vi "fp display engine resonance.vi"(7 "channel data in":sgl[][][](array[numeric]), 10 "Image Refs In":T1[](array[typedef]), 11 "DisplayRefsIn(generic class)":refnum<vi>[](array[refnum])) -> ()   [LabVIEW 2012]
doc: "SciScan 1.2 160622"
uses:
  <vilib>/vision/Image Controls.llb/IMAQ Image.ctl
  Custom Controls/MAIN Image panel reso tab Control type def.ctl
  Custom Controls/Image Types.ctl
  Custom Controls/Ch selector.ctl
  GFG/GFGbooleanGet.vi
  GFG/GFGfpRefGet.vi
  <vilib>/vision/NI_Vision_Development_Module.lvlib
  GFG/GFG library.lvlib
panel:
  in  "ROI colors":u32[](array[colorbox])=[6618880, 16716362, 16860, 16776793, 16750848, 16448250, 16716530, 9567230, 16764108, 7340212, 32639, 0, 13816530, 8421376, 8421631, 7171459, 6618880, 16716362, 16860, 16776793, 16750848, 16448250, 16716530, 9567230, 16764108, 7340212, 32639, 0, 13816530, 8421376, 8421631, 7171459, 6618880, 16716362, 16860, 16776793, 16750848, 16448250, 16716530, 9567230, 16764108, 7340212, 32639, 0, 13816530, 8421376, 8421631, 7171459, 6618880, 16716362, 16860, 16776793, 16750848, 16448250, 16716530, 9567230, 16764108, 7340212, 32639, 0, 13816530, 8421376, 8421631, 7171459, 6618880, 16716362, 16860, 16776793, 16750848, 16448250, 16716530, 9567230, 16764108, 7340212, 32639, 0, 13816530, 8421376, 8421631, 7171459, 6618880, 16716362, 16860, 16776793, 16750848, 16448250, 16716530, 9567230, 16764108, 7340212, 32639, 0, 13816530, 8421376, 8421631, 7171459, 6618880, 16716362, 16860, 16776793, 16750848, 16448250, 16716530, 9567230, 16764108, 7340212, 32639, 0, 13816530, 8421376, 8421631, 7171459, 6618880, 16716362, 16860, 16776793, 16750848, 16448250, 16716530, 9567230, 16764108, 7340212, 32639, 0, 13816530, 8421376, 8421631, 7171459, 6618880, 16716362, 16860, 16776793, 16750848, 16448250, 16716530, 9567230, 16764108, 7340212, 32639, 0, 13816530, 8421376, 8421631, 7171459, 6618880, 16716362, 16860, 16776793, 16750848, 16448250, 16716530, 9567230, 16764108, 7340212, 32639, 0, 13816530, 8421376, 8421631, 7171459, 6618880, 16716362, 16860, 16776793, 16750848, 16448250, 16716530, 9567230, 16764108, 7340212, 32639, 0, 13816530, 8421376, 8421631, 7171459, 6618880, 16716362, 16860, 16776793, 16750848, 16448250, 16716530, 9567230, 16764108, 7340212, 32639, 0, 13816530, 8421376, 8421631, 7171459, 6618880, 16716362, 16860, 16776793, 16750848, 16448250, 16716530, 9567230, 16764108, 7340212, 32639, 0, 13816530, 8421376, 8421631, 7171459, 6618880, 16716362, 16860, 16776793, 16750848, 16448250, 16716530, 9567230, 16764108, 7340212, 32639, 0, 13816530, 8421376, 8421631, 7171459, 6618880, 16716362, 16860, 16776793, 16750848, 16448250, 16716530, 9567230, 16764108, 7340212, 32639, 0, 13816530, 8421376, 8421631, 7171459, 6618880, 16716362, 16860, 16776793, 16750848, 16448250, 16716530, 9567230, 16764108, 7340212, 32639, 0, 13816530, 8421376, 8421631, 7171459, 6618880, 16716362, 16860, 16776793, 16750848, 16448250, 16716530, 9567230, 16764108, 7340212, 32639, 0, 13816530, 8421376, 8421631, 7171459, 6618880, 16716362, 16860, 16776793, 16750848, 16448250, 16716530, 9567230, 16764108, 7340212, 32639, 0, 13816530, 8421376, 8421631, 7171459, 6618880, 16716362, 16860, 16776793, 16750848, 16448250, 16716530, 9567230, 16764108, 7340212, 32639, 0, 13816530, 8421376, 8421631, 7171459, 6618880, 16716362, 16860, 16776793, 16750848, 16448250, 16716530, 9567230, 16764108, 7340212, 32639, 0, 13816530, 8421376, 8421631, 7171459, 6618880, 16716362, 16860, 16776793, 16750848, 16448250, 16716530, 9567230, 16764108, 7340212, 32639, 0, 13816530, 8421376, 8421631, 7171459, 6618880, 16716362, 16860, 16776793, 16750848, 16448250, 16716530, 9567230, 16764108, 7340212, 32639, 0, 13816530, 8421376, 8421631, 7171459, 6618880, 16716362, 16860, 16776793, 16750848, 16448250, 16716530, 9567230, 16764108, 7340212, 32639, 0, 13816530, 8421376, 8421631, 7171459, 6618880, 16716362, 16860, 16776793, 16750848, 16448250, 16716530, 9567230, 16764108, 7340212, 32639, 0, 13816530, 8421376, 8421631, 7171459, 6618880, 16716362, 16860, 16776793, 16750848, 16448250, 16716530, 9567230, 16764108, 7340212, 32639, 0, 13816530, 8421376, 8421631, 7171459]
  out "error out":errorcluster
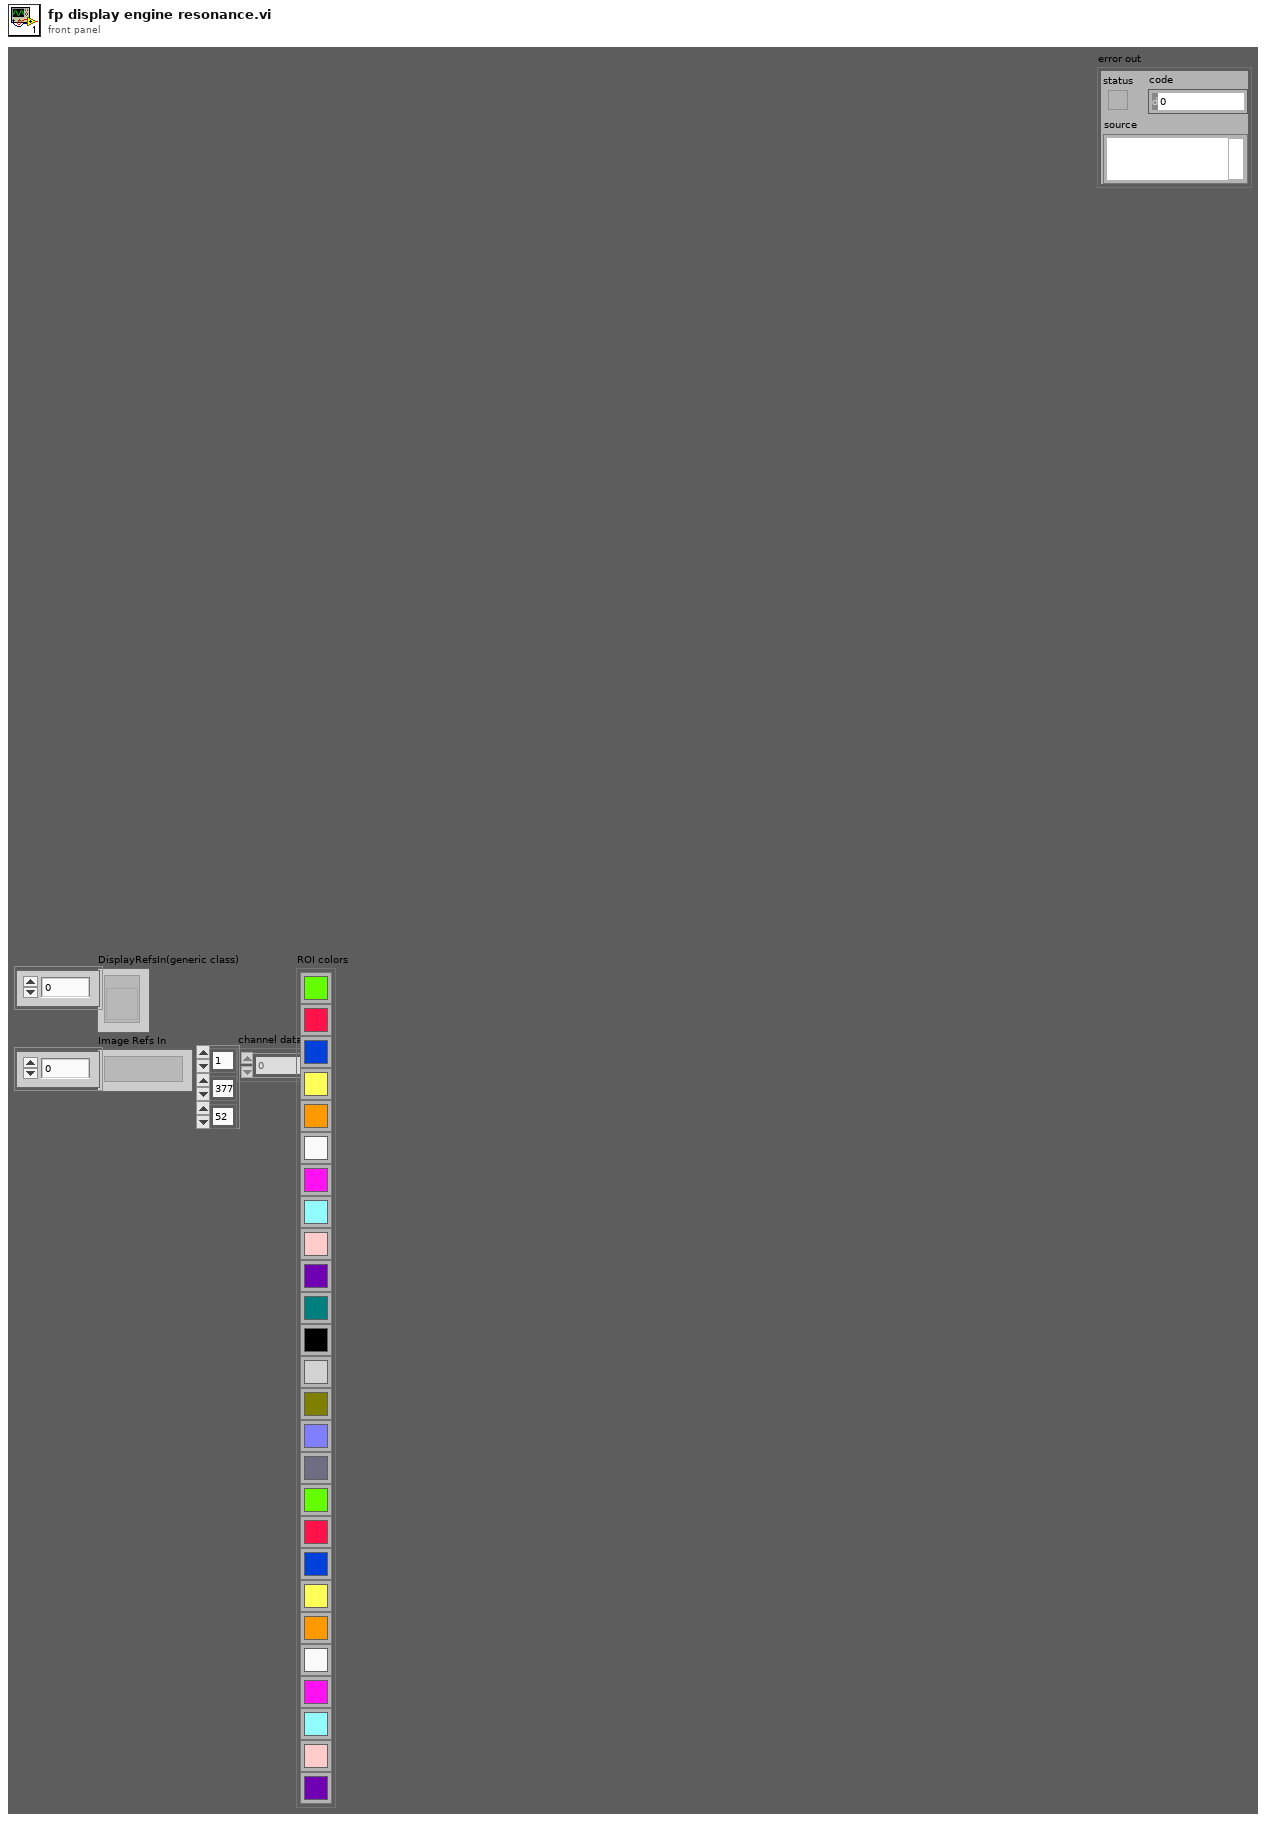
[diagram p1: front panel]
types:
  T1 = typedef "IMAQ Image.ctl" = refnum<image>
  T2 = typedef "MAIN Image panel reso tab Control type def.ctl" = enum32{"Channel 1", "Channel 2", "Channel 3", "Channel 4", "Channel 5", "all channels", "RGB overlay", "ROI", "arbitrary line scan"}
  T3 = enum32{"Channel 1", "Channel 2", "Channel 3", "Channel 4", "Channel 5", "all channels", "RGB overlay", "ROI", "arbitrary line scan"}
  T4 = typedef "Image Types.ctl" = enum16{"Frame Scan", "Line Scan", "RGB Overlay", "ROI", "All Channels Frame"}
  T5 = typedef "Ch selector.ctl" = enum16{"none", "Ch 1", "Ch 2", "Ch 3", "Ch 4"}
  T6 = typedef "Image Type" = u32
  T7 = cluster{"Global Rectangle":i32[], "Contours":cluster{"Contour Type":u32, "ROI Type":u32, "Points":i32[]}[]}
  T8 = typedef "ROI Descriptor" = cluster{"Global Rectangle":i32[], "Contours":cluster{"ID":enum32{"External", "Internal"}, "Type":u32, "Coordinates":i32[]}[]}
  T9 = cluster{"WaveformChartRef":refnum<vi>, "DigitalRef":refnum<vi>, "ArrayRef":refnum<vi>, "TabControlRef":refnum<vi>, "EnumRef":refnum<vi>, "RingRef":refnum<vi>, "BooleanRef":refnum<vi>, "KnobRef":refnum<vi>, "SlideRef":refnum<vi>, "PathRef":refnum<vi>, "StringRef":refnum<vi>, "ComboBox":refnum<vi>, "WaveformGraphRef":refnum<vi>}
  T10 = cluster{"Mean Value":sgl, "Standard Variation":sgl, "Minimal Value":sgl, "Maximal Value":sgl, "Area (calibrated)":sgl, "Area (pixels)":i32, "%":sgl}[]
  T11 = cluster{"Mean Value":sgl, "Standard Variation":sgl, "Minimal Value":sgl, "Maximal Value":sgl, "Area (calibrated)":sgl, "Area (pixels)":i32, "%":sgl}
  T12 = cluster{"Contour Type":u32, "ROI Type":u32, "Points":i32[]}[]
  T13 = cluster{"Starting Value":sgl, "Incremental Value":sgl, "Histogram":u32[]}
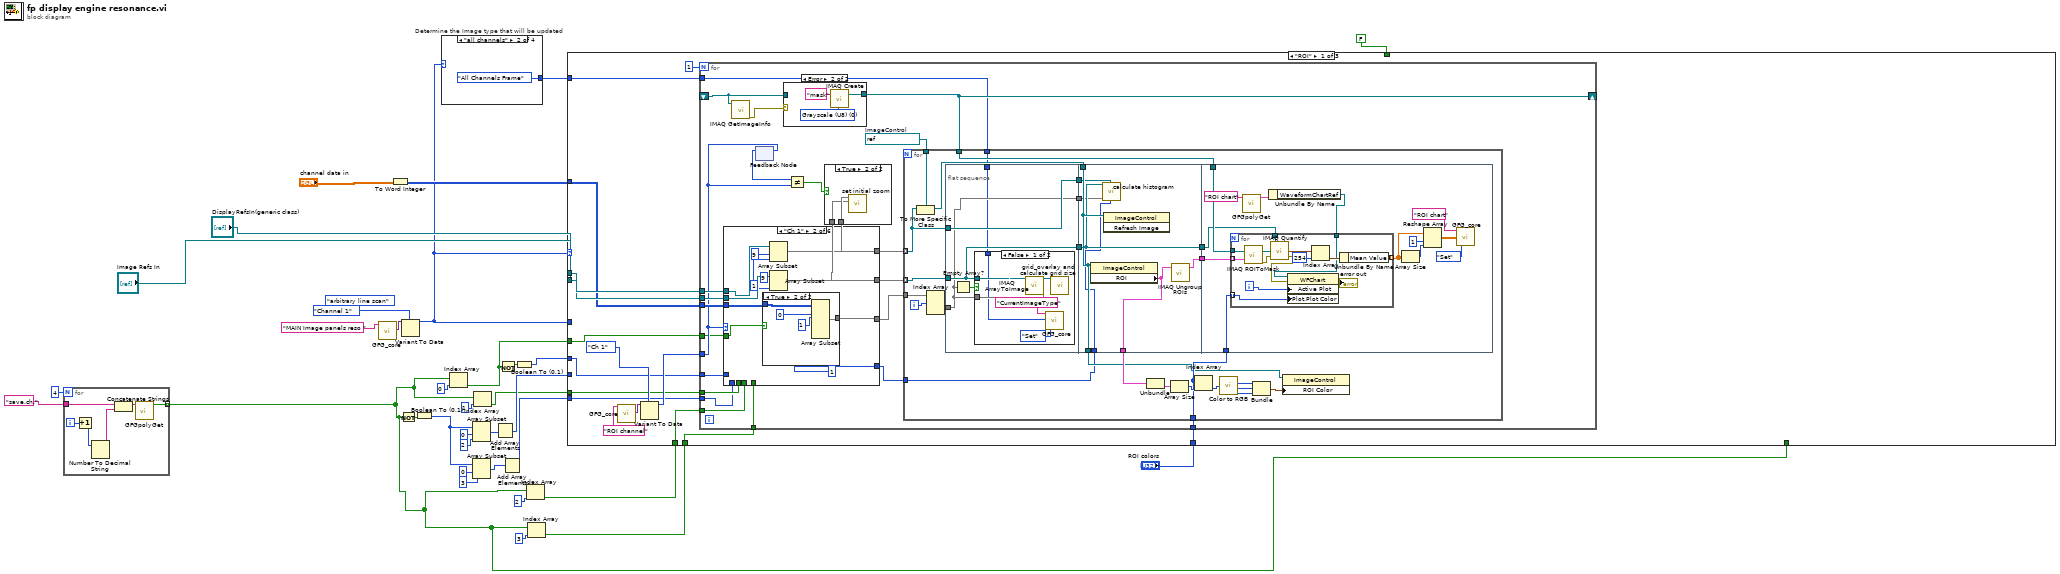
[diagram p0: block diagram]
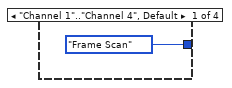
[diagram p2: hidden frame]
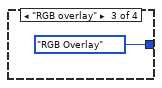
[diagram p3: hidden frame]
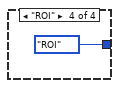
[diagram p4: hidden frame]
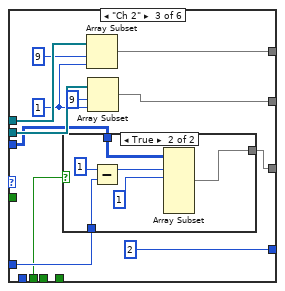
[diagram p9: hidden frame]
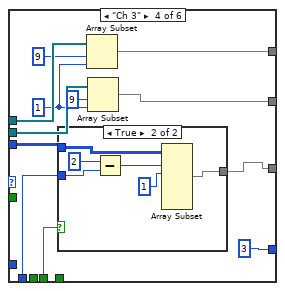
[diagram p11: hidden frame]
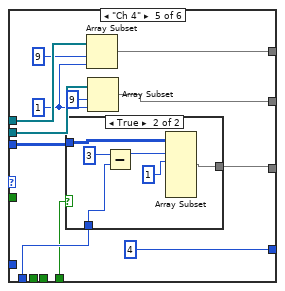
[diagram p13: hidden frame]
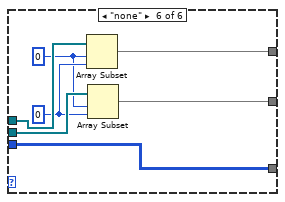
[diagram p15: hidden frame]
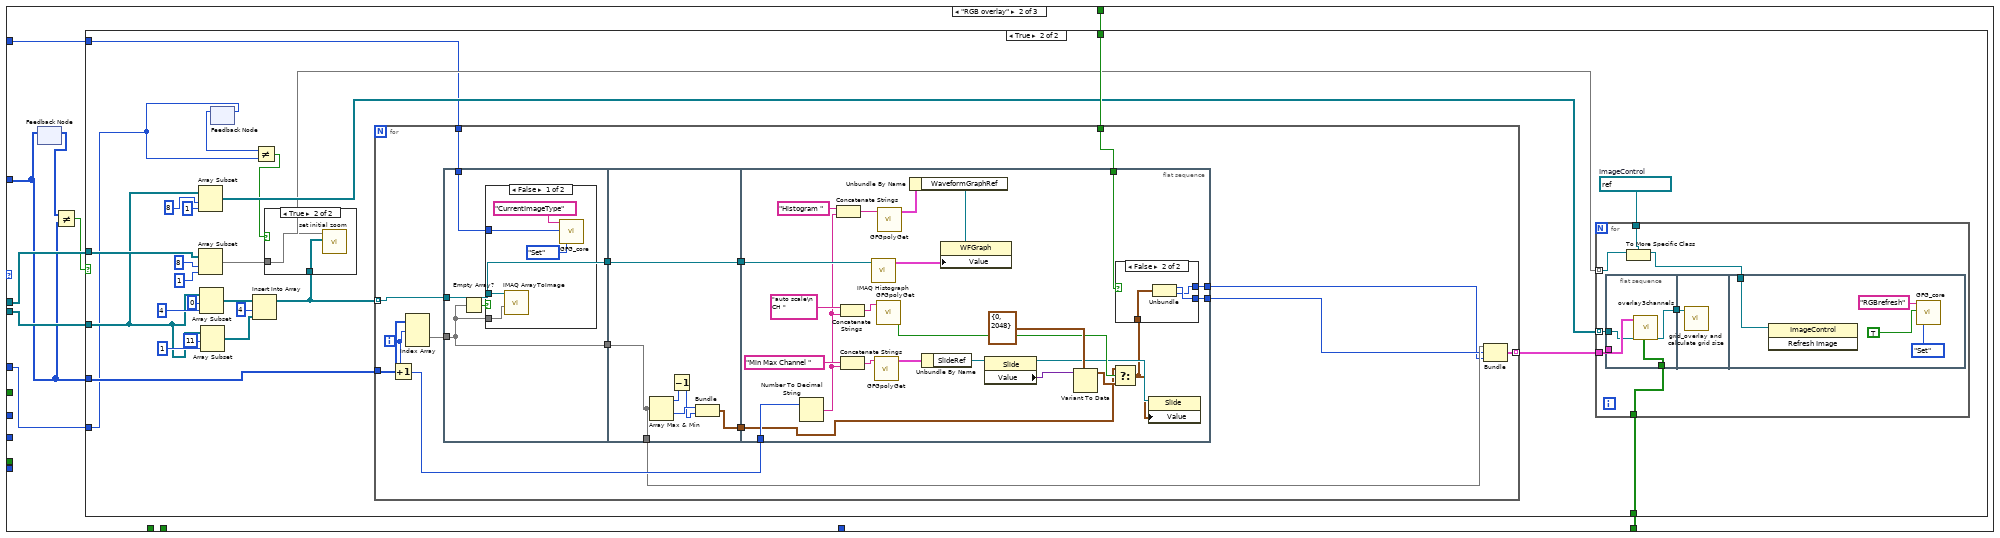
[diagram p17: hidden frame]
diagram:
  (unwired) T3."arbitrary line scan" ("MAIN Image panels")
  n1 = for {
    N: 4 -> [_]
    tunnel: "save.ch." ("Variable Name in") -> [w40]
    tunnel: [w39] -> w4 mode=indexing
    i -> [w38]
    n2 = Increment(x=w38) -> (x+1=w37:i32)
    n3 = Number To Decimal String(number=w37) -> (decimal integer string=w35:string)  [unwired: 1 in]
    n4 = Concatenate Strings(w40, w35) -> (w36:string)
    n5 = call-poly "GFGpolyGet.vi"("Variable Name in"=w36) -> ("Boolean Value OUT"=w39:bool)  [unwired: 9 in, 1 out]
  }
  n6 = call "GFG_core.vi"("Variable Name in"="MAIN Image panels reso ") -> ("Variant Out"=w34:variant)  [unwired: 12 in, 6 out]
  n7 = To Word Integer(number="channel data in") -> (16bit integer=w29:i16[][][])
  n8 = Not(x=w4) -> (.not. x?=w18:bool[])
  n9 = Variant To Data(type=MAIN_Image_panel_reso_tab_Control_type_def."Channel 1" ("MAIN Image panels reso"), Variant=w34) -> (data=w2:T2)  [unwired: 1 in, 1 out]
  n10 = Boolean To (0,1)(Boolean=w18) -> (0, 1=w19:i16[])
  n11 = case "Determine the Image type that will be updated" shown="\"all channels\"" w2 {
    tunnel: [Image_Types."Frame Scan" ("Image Types") Image_Types."All Channels Frame" ("Image Types") Image_Types."RGB Overlay" ("Image Types") Image_Types."ROI" ("Image Types")] -> w1
    frame "Channel 1".."Channel 4", Default {
    }
    frame "all channels" {
    }
    frame "RGB overlay" {
    }
    frame "ROI" {
    }
  }
  n12 = Index Array(array=w4, index=0) -> (element=w13:bool)
  n13 = Array Subset(array=w19, index=0, length=3) -> (w15:i16[])
  n14 = Array Subset(array=w19, index=0, length=2) -> (w17:i16[])
  n15 = Index Array(array=w4, index=1) -> (element=w9:bool)
  n16 = Add Array Elements(numeric array=w17) -> (sum=w16:i16)
  n17 = Not(x=w13) -> (.not. x?=w12:bool)
  n18 = Add Array Elements(numeric array=w15) -> (sum=w14:i16)
  n19 = Boolean To (0,1)(Boolean=w12) -> (0, 1=w11:i16)
  n20 = Index Array(array=w4, index=2) -> (element=w6:bool)
  n21 = Index Array(array=w4, index=3) -> (element=w5:bool)
  n22 = case shown="\"ROI\"" w2 {
    tunnel: w2 -> [_ w236 w357]
    tunnel: "DisplayRefsIn(generic class)" -> [w59 w243 w360]
    tunnel: "Image Refs In" -> [w58 w241 w359]
    tunnel: w29 -> [w57 w239 w358]
    tunnel: FALSE -> [_ w242 w355]
    tunnel: "ROI colors" -> [w53 _ _]
    tunnel: w13 -> [w51 _ w354]
    tunnel: w16 -> [_ _ w353]
    tunnel: w14 -> [w48 _ w352]
    tunnel: w11 -> [w49 _ w351]
    tunnel: w9 -> [w50 _ w350]
    tunnel: w6 -> [w47 _ w349]
    tunnel: w5 -> [w46 _ w348]
    tunnel: w4 -> [_ w237 _]
    tunnel: w1 -> [w45 w235 w347]
    frame "ROI" {
      n23 = call "GFG_core.vi"("Variable Name in"="ROI channel") -> ("Variant Out"=w55:variant)  [unwired: 12 in, 6 out]
      n24 = Variant To Data(type=Ch_selector."Ch 1" ("ROI channel"), Variant=w55) -> (data=w54:T5)  [unwired: 1 in, 1 out]
      n25 = for {
        N: 1 -> [_]
        tunnel: w59 -> [w81]
        tunnel: w58 -> [w80]
        tunnel: w57 -> [w79]
        tunnel: w54 -> [w76]
        shift-right: [w73] -> _
        shift-left: _ -> [w72]
        tunnel: w53 -> [w70]
        tunnel: w51 -> [w67]
        tunnel: w49 -> [w66]
        tunnel: w50 -> [w65]
        tunnel: w48 -> [w64]
        tunnel: w47 -> [w63]
        tunnel: w46 -> [w62]
        tunnel: w45 -> [w61]
        w78 = refnum<vi> refnum  # ImageControl
        n26 = case shown="\"Ch 1\"" w76 {
          tunnel: w81 -> [_ w98 w114 w132 w150 w163]
          tunnel: w80 -> [_ w99 w115 w133 w151 w164]
          tunnel: [_ w95 w111 w129 w147 w160] -> w68
          tunnel: [_ w94 w110 w128 w146 w159] -> w75
          tunnel: w79 -> [_ w91 w107 w124 w142 w158]
          tunnel: [_ w89 w106 w125 w143 w158] -> w82
          tunnel: [_ 1 ("length") 2 ("length") 3 ("length") 4 ("length") _] -> w69
          tunnel: w67 -> [_ w90 _ _ _ _]
          tunnel: w66 -> [_ _ w105 _ _ _]
          tunnel: w65 -> [_ _ w104 _ _ _]
          tunnel: w64 -> [_ _ _ w123 w141 _]
          tunnel: w63 -> [_ _ _ w122 _ _]
          tunnel: w62 -> [_ _ _ _ w140 _]
          frame Default {
          }
          frame "Ch 1" {
            w97 = 1 ("length")
            n27 = case shown="True" w90 {
              tunnel: w91 -> [_ w103]
              tunnel: [_ w101] -> w89
              frame False {
              }
              frame True {
                n28 = Array Subset(array=w103, index (dim 0)=0 ("index"), length (dim 0)=1 ("length")) -> (w101:i16[][][])  [unwired: 4 in]
              }
            }
            n29 = Array Subset(array=w98, index=9, length=w97) -> (w94:refnum<vi>[])
            n30 = Array Subset(array=w99, index=9, length=w97) -> (w95:T1[])
          }
          frame "Ch 2" {
            w113 = 1 ("length")
            n31 = case shown="True" w104 {
              tunnel: w107 -> [_ w119]
              tunnel: [_ w118] -> w106
              tunnel: w105 -> [_ w116]
              frame False {
              }
              frame True {
                n32 = Subtract(x=1 ("index"), y=w116) -> (x-y=w117:i32)
                n33 = Array Subset(array=w119, index (dim 0)=w117, length (dim 0)=1 ("length")) -> (w118:i16[][][])  [unwired: 4 in]
              }
            }
            n34 = Array Subset(array=w114, index=9, length=w113) -> (w110:refnum<vi>[])
            n35 = Array Subset(array=w115, index=9, length=w113) -> (w111:T1[])
          }
          frame "Ch 3" {
            w130 = 1 ("index")
            n36 = case shown="True" w122 {
              tunnel: w124 -> [_ w138]
              tunnel: [_ w137] -> w125
              tunnel: w123 -> [_ w135]
              frame False {
              }
              frame True {
                n37 = Subtract(x=2 ("index"), y=w135) -> (x-y=w136:i32)
                n38 = Array Subset(array=w138, index (dim 0)=w136, length (dim 0)=1 ("length")) -> (w137:i16[][][])  [unwired: 4 in]
              }
            }
            n39 = Array Subset(array=w132, index=9, length=w130) -> (w128:refnum<vi>[])
            n40 = Array Subset(array=w133, index=9, length=w130) -> (w129:T1[])
          }
          frame "Ch 4" {
            w149 = 1 ("index")
            n41 = case shown="True" w140 {
              tunnel: w142 -> [_ w156]
              tunnel: [_ w155] -> w143
              tunnel: w141 -> [_ w152]
              frame False {
              }
              frame True {
                n42 = Subtract(x=3 ("index"), y=w152) -> (x-y=w154:i32)
                n43 = Array Subset(array=w156, index (dim 0)=w154, length (dim 0)=1 ("length")) -> (w155:i16[][][])  [unwired: 4 in]
              }
            }
            n44 = Array Subset(array=w150, index=9, length=w149) -> (w146:refnum<vi>[])
            n45 = Array Subset(array=w151, index=9, length=w149) -> (w147:T1[])
          }
          frame "none" {
            w161 = 0 ("index")
            w162 = 0 ("length")
            n46 = Array Subset(array=w163, index=w161, length=w162) -> (w159:refnum<vi>[])
            n47 = Array Subset(array=w164, index=w161, length=w162) -> (w160:T1[])
          }
        }
        n48 = call "IMAQ GetImageInfo"("Image"=w72) -> ("error out"=w71:errorcluster)  [unwired: 3 in, 7 out]
        n49 = feedback-in #1(w76) -> ()
        n50 = feedback #1() -> (w77:T5)  [unwired: 1 in]
        n51 = case shown="Error" w71 {
          tunnel: [w83 w84] -> w73
          tunnel: w72 -> [w83 _]
          frame No Error {
          }
          frame Error {
            w85 = T6 0 items=["Grayscale (U8)", "Grayscale (I16)", "Grayscale (SGL)", "Complex (CSG)", "RGB (U32)", "HSL (U32)", "RGB (U64)"] ("Image Type")
            n52 = call "IMAQ Create"("Image Name"="mask", "Image Type"=w85) -> ("New Image"=w84:T1)  [unwired: 3 in, 1 out]
          }
        }
        n53 = Not Equal?(x=w77, y=w76) -> (x != y?=w74:bool)
        n54 = case shown="True" w74 {
          tunnel: w75 -> [_ w88]
          tunnel: w68 -> [_ w87]
          frame False {
          }
          frame True {
            n55 = call "set initial zoom.vi"("Image Refs In"=w87, "DisplayRefsIn(generic class)"=w88) -> ()  [unwired: 10 in]
          }
        }
        n56 = for {
          tunnel: w75 -> [w168] mode=indexing
          tunnel: w68 -> [w187] mode=indexing
          tunnel: w82 -> [w189]
          tunnel: w78 -> [w186]
          tunnel: w73 -> [w171]
          tunnel: w70 -> [w174]
          tunnel: w69 -> [w166]
          tunnel: w61 -> [w165]
          i -> [w184]
          n57 = To More Specific Class(target class=w186, reference=w168) -> (specific class reference=w185:refnum<vi>)  [unwired: 1 in, 1 out]
          n58 = Index Array(array=w189, index (dim 0)=w184) -> (element=w188:i16[][])  [unwired: 2 in]
          n59 = flat-sequence {
            tunnel: w188 -> [w191]
            tunnel: w187 -> [w193]
            tunnel: [w193] -> w172
            tunnel: [w192] -> w169
            tunnel: w168 -> [w192]
            tunnel: [w191] -> w167
            tunnel: w165 -> [w190]
            tunnel: w185 -> [w205]
            tunnel: [w207] -> w177
            tunnel: [w206] -> w175
            tunnel: [w203] -> w173
            tunnel: w172 -> [w203]
            tunnel: [w205] -> w170
            tunnel: w169 -> [w204]
            tunnel: w167 -> [w202]
            tunnel: w166 -> [w201]
            tunnel: w175 -> [w217]
            tunnel: w174 -> [w216]
            tunnel: w173 -> [w208]
            tunnel: w171 -> [w209]
            frame #0 {
              n60 = Empty Array?(array=w191) -> (empty?=w194:bool)
              n61 = case shown="False" w194 {
                tunnel: w193 -> [w200 _]
                tunnel: w191 -> [w199 _]
                tunnel: w190 -> [w195 _]
                frame False {
                  n62 = call "IMAQ ArrayToImage"("Image Pixels (I16)"=w199, "Image"=w200) -> ("Image Out"=w198:T1)  [unwired: 8 in, 1 out]
                  n63 = call "GFG_core.vi"("Variable Name in"="CurrentImageType", "Variant in"=w195, "Action"=enum16{"Init", "Set", "Get", "Clear"}."Set") -> ()  [unwired: 10 in, 7 out]
                  n64 = call "grid_overlay and calculate grid size.vi"("Image In"=w198) -> ()  [unwired: 10 in, 1 out]
                }
                frame True {
                }
              }
            }
            frame #1 {
              n65 = property class="ImageControl"(reference=w205) -> ("ROI"=w207:T7)  [unwired: 1 in, 2 out]
              n66 = call "calculate histogram.vi"("channel no."=w201, "Image Ctrl Ref (as generic class)"=w204, "Image Array"=w202, "Image"=w203) -> ()  [unwired: 8 in]
              n67 = invoke class="ImageControl" method="Refresh Image"(reference=w205) -> ()  [unwired: 2 in, 3 out]
              n68 = call "IMAQ Ungroup ROIs"("ROI Descriptor"=w207) -> ("ROI Descriptors out"=w206:T8[])  [unwired: 3 in, 1 out]
            }
            frame #2 {
              n69 = call-poly "GFGpolyGet.vi"("Variable Name in"="ROI chart") -> ("output cluster"=w211:T9)  [unwired: 9 in, 1 out]
              n70 = Unbundle By Name(w211) -> ("WaveformChartRef"=w210:refnum<vi>)
              n71 = for {
                tunnel: w208 -> [w234]
                tunnel: w217 -> [w228] mode=indexing
                tunnel: [w230] -> w220 mode=indexing
                tunnel: w209 -> [w227]
                tunnel: w216 -> [w224] mode=indexing
                tunnel: w210 -> [w223]
                i -> [w225]
                n72 = call "IMAQ ROIToMask"("ROI Descriptor"=w228, "Image"=w227) -> ("error out"=w222:errorcluster, "Image Out"=w229:T1)  [unwired: 4 in, 1 out]
                n73 = call "IMAQ Quantify"("error in (no error)"=w222, "Image Mask"=w229, "Image"=w234) -> ("error out"=w221:errorcluster, "Region Reports"=w233:T10)  [unwired: 1 out]
                n74 = property on="Property Node" class="WFChart"(reference=w223, error in=w221, "Active Plot"=w225, "Plot.Plot Color"=w224) -> (error out=→"error out":errorcluster)  [unwired: 1 out]
                n75 = Index Array(array=w233, index=254) -> (element=w231:T11)
                n76 = Unbundle By Name(w231) -> ("Mean Value"=w230:sgl)
              }
              n77 = Array Size(array=w220) -> (size(s)=w219:i32)
              n78 = Reshape Array(w220, 1 ("dimension size"), w219) -> (w214:sgl[][])
              n79 = call "GFG_core.vi"("Variable Name in"="ROI chart", "Variant in"=w214, "Action"=enum16{"Init", "Set", "Get"}."Set") -> ()  [unwired: 10 in, 7 out]
            }
          }
          n80 = Unbundle(w177) -> ("Contours"=w182:T12)  [unwired: 1 out]
          n81 = Array Size(array=w182) -> (size(s)=w183:i32)
          n82 = Index Array(array=w174, index=w183) -> (element=w178:u32)
          n83 = call <vilib>:"Color to RGB.vi"("Color"=w178) -> ("R"=w179:u8, "G"=w180:u8, "B"=w181:u8)  [unwired: 1 out]
          n84 = Bundle("R"=w179, "G"=w180, "B"=w181) -> (w176:cluster{"R":u8, "G":u8, "B":u8})  [unwired: 1 in]
          n85 = property class="ImageControl"(reference=w170, "ROI Color"=w176) -> ()  [unwired: 1 in, 2 out]
        }
      }
    }
    frame "RGB overlay" {
      n86 = feedback-in #2(w239) -> ()
      n87 = feedback #2() -> (w240:i16[][][])  [unwired: 1 in]
      n88 = Not Equal?(x=w240, y=w239) -> (x != y?=w238:bool)
      n89 = case shown="True" w238 {
        tunnel: w243 -> [_ w268]
        tunnel: w239 -> [_ w267]
        tunnel: w242 -> [_ w266]
        tunnel: w241 -> [_ w252]
        tunnel: w237 -> [_ w248]
        tunnel: w236 -> [_ w246]
        tunnel: w235 -> [_ w244]
        frame False {
        }
        frame True {
          w255 = refnum<vi> refnum  # ImageControl
          n90 = Array Subset(array=w252, index=8, length=1) -> (w259:T1[])
          n91 = Array Subset(array=w268, index=8, length=1) -> (w256:refnum<vi>[])
          n92 = Array Subset(array=w252, index=0, length=4) -> (w257:T1[])
          n93 = Array Subset(array=w252, index=11, length=1) -> (w249:T1[])
          n94 = feedback #3() -> (w247:T2)  [unwired: 1 in]
          n95 = feedback-in #3(w246) -> ()
          n96 = Insert Into Array(array=w257, index=4, new element=w249) -> (w251:T1[])
          n97 = Not Equal?(x=w247, y=w246) -> (x != y?=w245:bool)
          n98 = case shown="True" w245 {
            tunnel: w256 -> [_ w270]
            tunnel: w251 -> [_ w269]
            frame False {
            }
            frame True {
              n99 = call "set initial zoom.vi"("Image Refs In"=w269, "DisplayRefsIn(generic class)"=w270) -> ()  [unwired: 10 in]
            }
          }
          n100 = for {
            tunnel: w251 -> [w299] mode=indexing
            tunnel: w267 -> [w301]
            tunnel: w266 -> [w292]
            tunnel: [w288] -> w258 mode=indexing
            tunnel: w244 -> [w287]
            i -> [w296]
            n101 = Increment(x=w296) -> (x+1=w294:i32)
            n102 = Index Array(array=w301, index (dim 0)=w296) -> (element=w300:i16[][])  [unwired: 2 in]
            n103 = flat-sequence {
              tunnel: w300 -> [w303]
              tunnel: w299 -> [w304]
              tunnel: [w304] -> w297
              tunnel: [w303] -> w295
              tunnel: w287 -> [w302]
              tunnel: [w316] -> w298
              tunnel: w297 -> [w316]
              tunnel: w295 -> [w311]
              tunnel: [w314] -> w293
              tunnel: [w311] -> w291
              tunnel: w298 -> [w335]
              tunnel: w294 -> [w334]
              tunnel: w293 -> [w322]
              tunnel: w292 -> [w317]
              tunnel: [w319] -> w289
              tunnel: [w318] -> w290
              frame #0 {
                n104 = Empty Array?(array=w303) -> (empty?=w305:bool)
                n105 = case shown="False" w305 {
                  tunnel: w304 -> [w310 _]
                  tunnel: w303 -> [w309 _]
                  tunnel: w302 -> [w306 _]
                  frame False {
                    n106 = call "IMAQ ArrayToImage"("Image Pixels (I16)"=w309, "Image"=w310) -> ()  [unwired: 8 in, 2 out]
                    n107 = call "GFG_core.vi"("Variable Name in"="CurrentImageType", "Variant in"=w306, "Action"=enum16{"Init", "Set", "Get", "Clear"}."Set") -> ()  [unwired: 10 in, 7 out]
                  }
                  frame True {
                  }
                }
              }
              frame #1 {
                n108 = Array Max & Min(array=w311) -> (max value=w315:i16, min value=w313:i16)  [unwired: 2 out]
                n109 = Decrement(x=w315) -> (x-1=w312:i16)
                n110 = Bundle(w313, w312) -> (w314:cluster{i16, i16})  [unwired: 1 in]
              }
              frame #2 {
                n111 = Number To Decimal String(number=w334) -> (decimal integer string=w329:string)  [unwired: 1 in]
                n112 = Concatenate Strings("Histogram " ("string"), w329) -> (w337:string)
                n113 = Concatenate Strings("auto scale\n      CH " ("Variable Name in"), w329) -> (w332:string)
                n114 = Concatenate Strings("Min Max Channel " ("Variable Name in"), w329) -> (w320:string)
                n115 = call "IMAQ Histograph"("Image"=w335) -> ("Histogram Graph"=w340:T13)  [unwired: 7 in, 3 out]
                n116 = call-poly "GFGpolyGet.vi"("Variable Name in"=w320) -> ("output cluster"=w331:T9)  [unwired: 9 in, 1 out]
                n117 = call-poly "GFGpolyGet.vi"("Variable Name in"=w332) -> ("Boolean Value OUT"=w325:bool)  [unwired: 9 in, 1 out]
                n118 = call-poly "GFGpolyGet.vi"("Variable Name in"=w337) -> ("output cluster"=w338:T9)  [unwired: 9 in, 1 out]
                n119 = Unbundle By Name(w338) -> ("WaveformGraphRef"=w339:refnum<vi>)
                n120 = Unbundle By Name(w331) -> ("SlideRef"=w328:refnum<vi>)
                n121 = property class="WFGraph"(reference=w339, "Value"=w340) -> ()  [unwired: 1 in, 2 out]
                n122 = property class="Slide"(reference=w328) -> (reference out=w323:refnum<vi>, "Value"=w327:variant)  [unwired: 1 in, 1 out]
                n123 = Variant To Data(type=cluster{i32, i32} {0, 2048} ("channel1"), Variant=w327) -> (data=w324:cluster{i32, i32})  [unwired: 1 in, 1 out]
                n124 = Select(t=w322, s=w325, f=w324) -> (s? t:f=w321:cluster{i32, i32})
                n125 = case shown="False" w317 {
                  tunnel: w321 -> [w343 w346]
                  tunnel: [w342 w344] -> w319
                  tunnel: [w341 w345] -> w318
                  frame True {
                    n126 = Unbundle(w343) -> (w342:i32, w341:i32)
                  }
                  frame False {
                    n127 = Unbundle(w346) -> (w345:i32, w344:i32)
                  }
                }
                n128 = property class="Slide"(reference=w323, "Value"=w321) -> ()  [unwired: 1 in, 2 out]
              }
            }
            n129 = Bundle(w291, w290, w289) -> (w288:cluster{i16[][], i32, i32})  [unwired: 1 in]
          }
          n130 = for {
            tunnel: w259 -> [w277] mode=indexing
            tunnel: w258 -> [w276]
            tunnel: w256 -> [w275] mode=indexing
            tunnel: w255 -> [w274]
            tunnel: w248 -> [w272]
            n131 = flat-sequence {
              tunnel: w277 -> [w279]
              tunnel: w276 -> [w281]
              tunnel: w272 -> [w280]
              tunnel: [w278] -> w271
              tunnel: w271 -> [w282]
              tunnel: w273 -> [w286]
              frame #0 {
                n132 = call "overlay3channels.vi"("active channels"=w280, "RGB Overlay"=w279, "Array"=w281) -> ("RGB Image Out"=w278:T1)  [unwired: 8 in]
              }
              frame #1 {
                n133 = call "grid_overlay and calculate grid size.vi"("Image In"=w282) -> ()  [unwired: 10 in, 1 out]
              }
              frame #2 {
                n134 = invoke class="ImageControl" method="Refresh Image"(reference=w286) -> ()  [unwired: 2 in, 3 out]
                n135 = call "GFG_core.vi"("Variable Name in"="RGBrefresh", "Variant in"=TRUE, "Action"=enum16{"Init", "Set", "Get"}."Set") -> ()  [unwired: 10 in, 7 out]
              }
            }
            n136 = To More Specific Class(target class=w274, reference=w275) -> (specific class reference=w273:refnum<vi>)  [unwired: 1 in, 1 out]
          }
        }
      }
    }
    frame Default {
      n137 = for {
        N: 1 -> [_]
        tunnel: w360 -> [w380]
        tunnel: w359 -> [w379]
        tunnel: w358 -> [w378]
        tunnel: w357 -> [w373]
        tunnel: w355 -> [w375]
        shift-right: [w373] -> _
        shift-left: _ -> [w372]
        tunnel: w354 -> [w370]
        tunnel: w353 -> [w369]
        tunnel: w352 -> [w368]
        tunnel: w351 -> [w367]
        tunnel: w350 -> [w366]
        tunnel: w349 -> [w365]
        tunnel: w348 -> [w364]
        tunnel: w347 -> [w361]
        n138 = case shown="\"Channel 1\"" w373 {
          tunnel: w380 -> [_ w391 w405 w422 w439]
          tunnel: w379 -> [_ w392 w406 w423 w440]
          tunnel: [_ w388 w402 w419 w436] -> w374
          tunnel: [_ w387 w401 w418 w435] -> w377
          tunnel: w378 -> [_ w386 w400 w416 w433]
          tunnel: [_ w385 w399 w415 w432] -> w381
          tunnel: w370 -> [_ w384 _ _ _]
          tunnel: w369 -> [_ _ _ w414 _]
          tunnel: w368 -> [_ _ _ _ w431]
          tunnel: w367 -> [_ _ w398 _ _]
          tunnel: w366 -> [_ _ w397 _ _]
          tunnel: w365 -> [_ _ _ w413 _]
          tunnel: w364 -> [_ _ _ _ w430]
          frame Default {
          }
          frame "Channel 1" {
            w389 = 4 ("index")
            w390 = 1 ("length")
            n139 = case shown="True" w384 {
              tunnel: w386 -> [_ w396]
              tunnel: [_ w394] -> w385
              frame False {
              }
              frame True {
                n140 = Array Subset(array=w396, index (dim 0)=0 ("index"), length (dim 0)=1 ("length")) -> (w394:i16[][][])  [unwired: 4 in]
              }
            }
            n141 = Array Subset(array=w391, index=w389, length=w390) -> (w387:refnum<vi>[])
            n142 = Array Subset(array=w392, index=w389, length=w390) -> (w388:T1[])
          }
          frame "Channel 2" {
            w403 = 5 ("index")
            w404 = 1 ("length")
            n143 = case shown="False" w397 {
              tunnel: w400 -> [_ w410]
              tunnel: [_ w409] -> w399
              tunnel: w398 -> [_ w407]
              frame False {
              }
              frame True {
                n144 = Subtract(x=1 ("index"), y=w407) -> (x-y=w408:i32)
                n145 = Array Subset(array=w410, index (dim 0)=w408, length (dim 0)=1 ("length")) -> (w409:i16[][][])  [unwired: 4 in]
              }
            }
            n146 = Array Subset(array=w406, index=w403, length=w404) -> (w402:T1[])
            n147 = Array Subset(array=w405, index=w403, length=w404) -> (w401:refnum<vi>[])
          }
          frame "Channel 3" {
            w420 = 1 ("index")
            w421 = 6 ("index")
            n148 = case shown="True" w413 {
              tunnel: 2 ("index") -> [_ w428]
              tunnel: w416 -> [_ w427]
              tunnel: [_ w426] -> w415
              tunnel: w414 -> [_ w424]
              frame False {
              }
              frame True {
                n149 = Subtract(x=w428, y=w424) -> (x-y=w425:i32)
                n150 = Array Subset(array=w427, index (dim 0)=w425, length (dim 0)=1 ("length")) -> (w426:i16[][][])  [unwired: 4 in]
              }
            }
            n151 = Array Subset(array=w422, index=w421, length=w420) -> (w418:refnum<vi>[])
            n152 = Array Subset(array=w423, index=w421, length=w420) -> (w419:T1[])
          }
          frame "Channel 4" {
            w437 = 7 ("index")
            w438 = 1 ("index")
            n153 = case shown="True" w430 {
              tunnel: 3 ("index") -> [_ w445]
              tunnel: w433 -> [_ w444]
              tunnel: [_ w443] -> w432
              tunnel: w431 -> [_ w441]
              frame False {
              }
              frame True {
                n154 = Subtract(x=w445, y=w441) -> (x-y=w442:i32)
                n155 = Array Subset(array=w444, index (dim 0)=w442, length (dim 0)=1 ("length")) -> (w443:i16[][][])  [unwired: 4 in]
              }
            }
            n156 = Array Subset(array=w439, index=w437, length=w438) -> (w435:refnum<vi>[])
            n157 = Array Subset(array=w440, index=w437, length=w438) -> (w436:T1[])
          }
        }
        n158 = Not Equal?(x=w372, y=w373) -> (x != y?=w376:bool)
        n159 = for {
          tunnel: w377 -> [w450] mode=indexing
          tunnel: w374 -> [w452] mode=indexing
          tunnel: w381 -> [w457]
          tunnel: w373 -> [w456]
          tunnel: w375 -> [_]
          tunnel: [w449] -> w371
          tunnel: w361 -> [w447]
          i -> [w449]
          n160 = Increment(x=w449) -> (x+1=w455:i32)
          n161 = Index Array(array=w457, index (dim 0)=w449) -> (element=w448:i16[][])  [unwired: 2 in]
          n162 = flat-sequence {
            tunnel: w448 -> [w459]
            tunnel: w452 -> [w460]
            tunnel: [w460] -> w454
            tunnel: [w459] -> w453
            tunnel: w447 -> [w458]
            tunnel: w454 -> [w470]
            tunnel: w453 -> [w472]
            tunnel: w451 -> [w471]
            tunnel: w450 -> [w469]
            frame #0 {
              n163 = Empty Array?(array=w459) -> (empty?=w461:bool)
              n164 = case shown="False" w461 {
                tunnel: w460 -> [w467 _]
                tunnel: w459 -> [w466 _]
                tunnel: w458 -> [w462 _]
                frame False {
                  n165 = call "IMAQ ArrayToImage"("Image Pixels (I16)"=w466, "Image"=w467) -> ("Image Out"=w465:T1)  [unwired: 8 in, 1 out]
                  n166 = call "grid_overlay and calculate grid size.vi"("Image In"=w465) -> ()  [unwired: 10 in, 1 out]
                  n167 = call "GFG_core.vi"("Variable Name in"="CurrentImageType", "Variant in"=w462, "Action"=enum16{"Init", "Set", "Get", "Clear"}."Set") -> ()  [unwired: 10 in, 7 out]
                }
                frame True {
                }
              }
            }
            frame #1 {
              n168 = call "calculate histogram.vi"("channel no."=w471, "Image Ctrl Ref (as generic class)"=w469, "Image Array"=w472, "T for reso F for galvo"=TRUE, "Image"=w470) -> ()  [unwired: 7 in]
            }
          }
          n169 = case shown="\"Channel 1\", Default" w456 {
            tunnel: [1 2 3 4 w477] -> w451
            tunnel: w455 -> [_ _ _ _ w477]
            frame "Channel 1", Default {
            }
            frame "Channel 2" {
            }
            frame "Channel 3" {
            }
            frame "Channel 4" {
            }
            frame "all channels" {
            }
          }
        }
        n170 = First Call?() -> (First Call?: T/F=w362:bool)
        n171 = Or(x=w376, y=w362) -> (x .or. y?=w363:bool)
        n172 = case shown="True" w363 {
          tunnel: w377 -> [_ w383]
          tunnel: w374 -> [_ w382]
          tunnel: w371 -> [_ _]
          frame False {
          }
          frame True {
            n173 = call "set initial zoom.vi"("Image Refs In"=w382, "DisplayRefsIn(generic class)"=w383) -> ()  [unwired: 10 in]
          }
        }
      }
    }
  }
